vi "DAQ Initialize.vi"(8 "error in (no error)":errorcluster, 11 "Acquisition and Logging Configuration":T1={"Data Rate (Hz)"=1.0, "Samples per Read"=0, "Number of Reads to Save"=0, "Data File Name"="", "TDMS Properties"=[], "Number of Channels"=4, "Channel Scale Array"=[0.0, 0.0, 0.0, 0.0], "Channel Names"=[], "Trigger - RMS Value"=0.0, "Trigger - Channel"=0, "Trigger - Time (Minute)"=0, "Enable RMS Trigger"=FALSE, "Enable Time Trigger"=FALSE, "Always Log"=FALSE}) -> (0 "error out":errorcluster, 3 "DAQmx Task Name":refnum<k21>)   [LabVIEW 2013]
uses:
  Tests/Untitled Project 2/controls/Acquisition and Logging Configuration.ctl
  Tests/Untitled Project 2/controls/TDMS Properties.ctl
  <vilib>/DAQmx/create/channels.llb/DAQmx Create Channel (AI-Voltage-Basic).vi
  <vilib>/DAQmx/configure/timing.llb/DAQmx Timing (Sample Clock).vi
  <resource>/objmgr/daqmx.rc
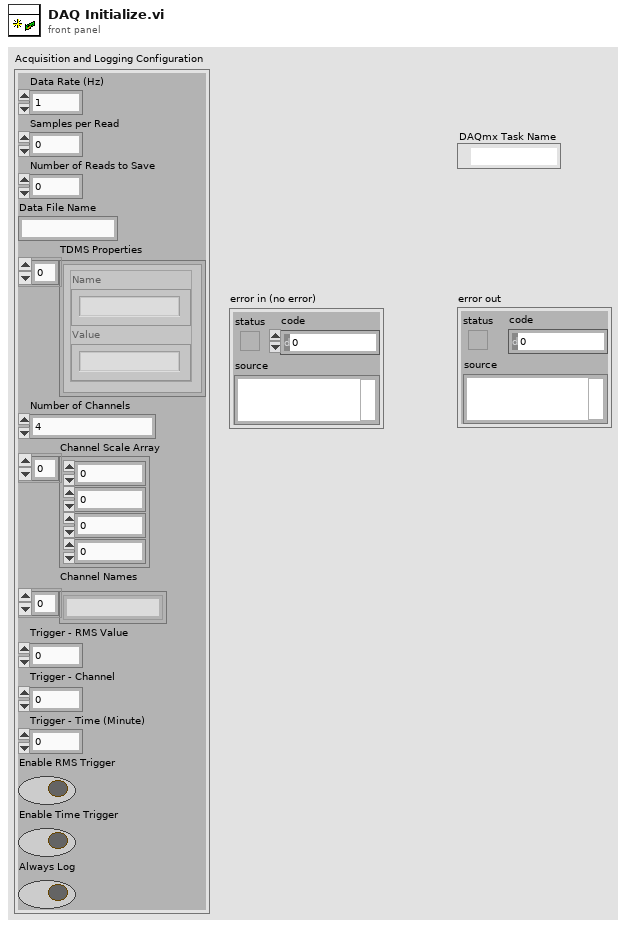
[diagram p1: front panel]
types:
  T1 = typedef "Acquisition and Logging Configuration.ctl" = cluster{"Data Rate (Hz)":dbl, "Samples per Read":i32, "Number of Reads to Save":i32, "Data File Name":string, "TDMS Properties":T2[], "Number of Channels":i32, "Channel Scale Array":dbl[], "Channel Names":string[], "Trigger - RMS Value":dbl, "Trigger - Channel":i32, "Trigger - Time (Minute)":i32, "Enable RMS Trigger":bool, "Enable Time Trigger":bool, "Always Log":bool}
  T2 = typedef "TDMS Properties.ctl" = cluster{"Name":string, "Value":string}
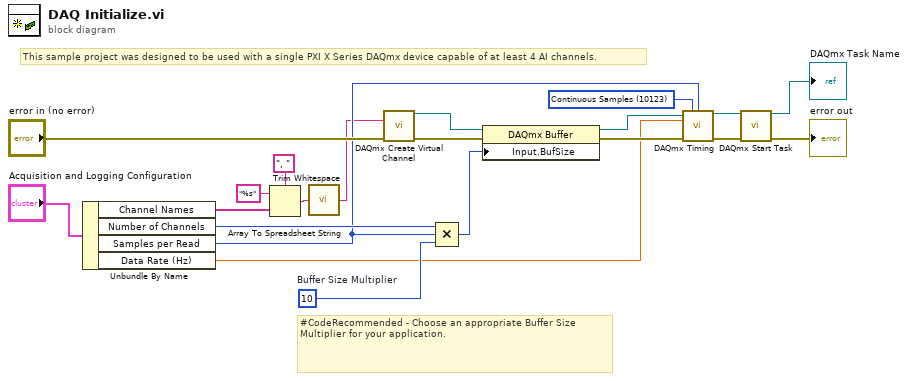
[diagram p0: block diagram]
diagram:
  w7 = 10123 items=["Finite Samples"=10178, "Continuous Samples"=10123, "Hardware Timed Single Point"=12522] ("sample mode")
  w13 = 10  # Buffer Size Multiplier
  # "This sample project was designed to be used with a single PXI X Series DAQmx device capable of at least 4 AI channels."
  # "#CodeRecommended - Choose an appropriate Buffer Size Multiplier for your application."
  n1 = Unbundle By Name("Acquisition and Logging Configuration") -> ("Channel Names"=w19:string[], "Number of Channels"=w14:i32, "Samples per Read"=w6:i32, "Data Rate (Hz)"=w5:dbl)
  n2 = Array To Spreadsheet String(delimiter (Tab)=", ", array=w19, 3:"%s" ("format string")) -> (spreadsheet string=w2:string)
  n3 = call <vilib>:"Trim Whitespace.vi"("string"=w2) -> ("trimmed string"=w1:string)  [unwired: 1 in]
  n4 = call-poly <vilib>:"DAQmx Create Virtual Channel.vi"("physical channels"=w1, "error in"="error in (no error)") -> ("task out"=w15:refnum<k21>, "error out"=w16:errorcluster)  [unwired: 12 in]
  n5 = Compound Arithmetic op=MULTIPLY(w14, w6, w13) -> (w12:i32)
  n6 = property class="DAQmx Buffer"(reference=w15, error in=w16, "Input.BufSize"=w12) -> (reference out=w8:refnum<k21>, error out=w9:errorcluster)
  n7 = call-poly <vilib>:"DAQmx Timing.vi"("task/channels in"=w8, "sample mode"=w7, "samples per channel"=w6, "rate"=w5, "error in"=w9) -> ("task out"=w10:refnum<k21>, "error out"=w11:errorcluster)  [unwired: 9 in]
  n8 = call <vilib>:"DAQmx Start Task.vi"("task/channels in"=w10, "error in"=w11) -> ("task out"=→"DAQmx Task Name":refnum<k21>, "error out"=→"error out":errorcluster)  [unwired: 12 in]
